vi "Clear Commands.vi"(8 "error in (no error)":errorcluster, 11 "ITX Commands in":refnum<class "ITX Commands.lvclass">) -> (0 "error out":errorcluster, 3 "ITX Commands out":refnum<class "ITX Commands.lvclass">)   [LabVIEW 2019, in "ITX Commands.lvclass"]
uses:
  ITX Commands.lvclass
  ITX Commands.lvclass/ITX Commands.ctl
panel:
  out "Command String":string
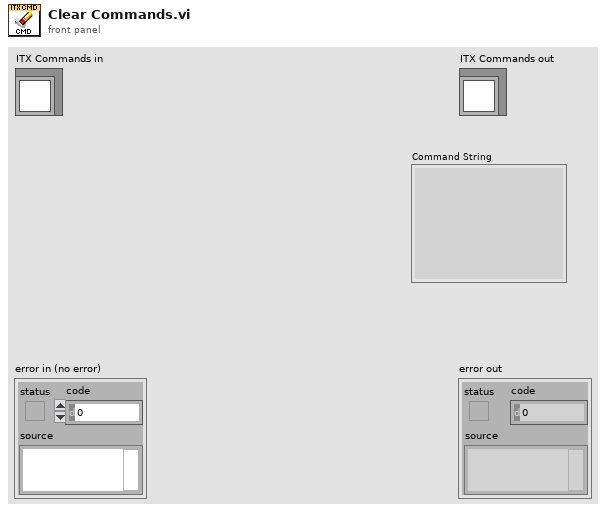
[diagram p1: front panel]
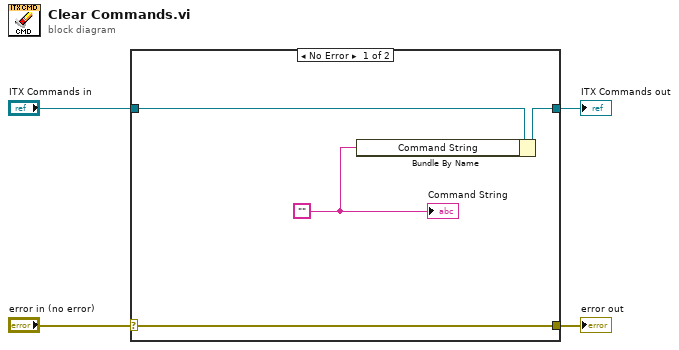
[diagram p0: block diagram]
diagram:
  n1 = case shown="No Error" "error in (no error)" {
    selector: "error in (no error)" -> [w7 w10]
    tunnel: [w7 w10] -> w3
    tunnel: [w8 w9] -> w1
    tunnel: "ITX Commands in" -> [w6 w9]
    frame No Error {
      w5 = ""
      n2 = Bundle By Name(cluster=w6, "Command String"=w5) -> (w8:refnum<class "ITX Commands.lvclass">)
      "Command String" <- w5
    }
    frame Error {
    }
  }
  "error out" <- w3
  "ITX Commands out" <- w1
